vi "DequeueExperiment.vi"(0 "object in":refnum<class "Experiment.lvclass">, 5 "error in (no error)":errorcluster) -> (11 "QueueEmpty?":bool, 14 "object out":refnum<class "Experiment.lvclass">, 15 "Message":string, 16 "Message Data":variant, 17 "Wait Command":bool, 19 "error out":errorcluster)   [LabVIEW 2021, in "Experiment.lvclass"]
uses:
  Experiment.lvclass
  Experiment.lvclass/Experiment.ctl
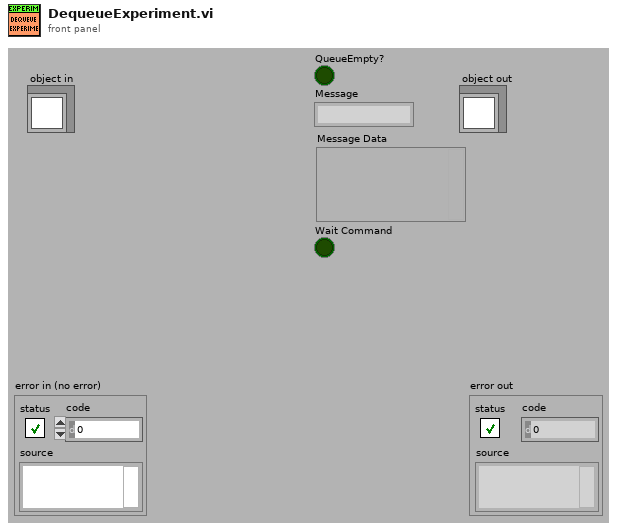
[diagram p1: front panel]
types:
  T1 = cluster{"Message":string, "Message Data":variant, "Wait Command":bool}
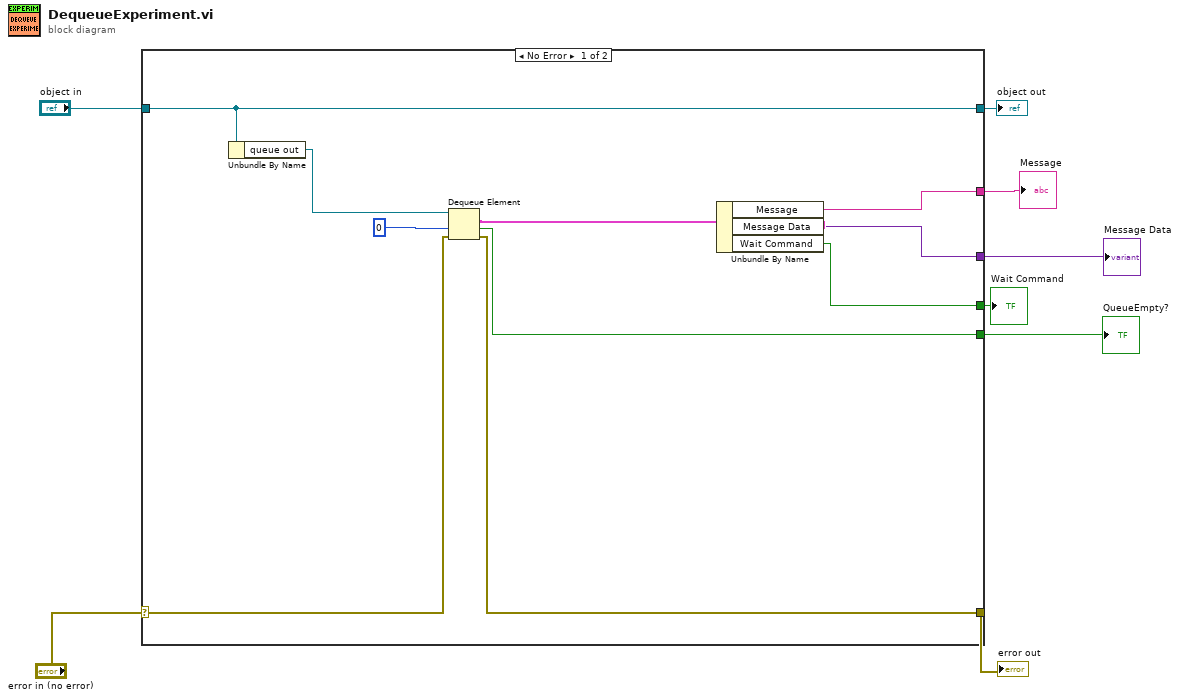
[diagram p0: block diagram]
diagram:
  n1 = case shown="No Error" "error in (no error)" {
    selector: "error in (no error)" -> [w16 w20]
    tunnel: [w15 w20] -> w7
    tunnel: [w18 w19] -> w5
    tunnel: "object in" -> [w18 w19]
    tunnel: [w14 _] -> w4
    tunnel: [w11 _] -> w3
    tunnel: [w10 _] -> w2
    tunnel: [w9 _] -> w1
    frame No Error {
      n2 = Unbundle By Name(w18) -> ("queue out"=w17:refnum<queue>)
      n3 = Dequeue Element(queue=w17, timeout in ms (-1)=0, error in (no error)=w16) -> (element=w12:T1, timed out?=w14:bool, error out=w15:errorcluster)  [unwired: 1 out]
      n4 = Unbundle By Name(w12) -> ("Message"=w11:string, "Message Data"=w10:variant, "Wait Command"=w9:bool)
    }
    frame Error {
    }
  }
  "error out" <- w7
  "object out" <- w5
  "QueueEmpty?" <- w4
  "Message" <- w3
  "Message Data" <- w2
  "Wait Command" <- w1
